vi "Example Threshold - IlluminanceReached Callback.vi"(4 "IlluminanceReached":refnum<user-event>, 5 "Event Data":cluster{"sender":refnum<k24>, "illuminance":i64}, 6 "Control Ref":refnum<k24>, 7 "Event Common Data":T1) -> ()   [LabVIEW 2013]
uses:
  C:/tf/play/labview/Tinkerforge.dll
  Tinkerforge.dll
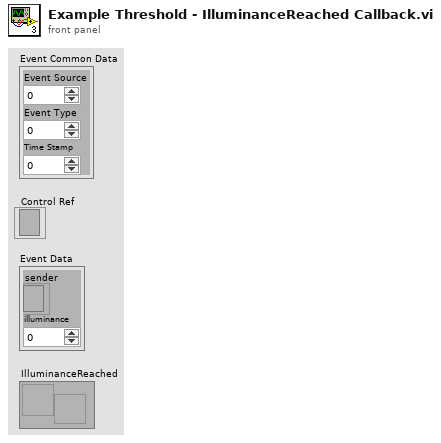
[diagram p1: front panel]
types:
  T1 = cluster{"Event Source":i32, "Event Type":u32, "Time Stamp":u32}
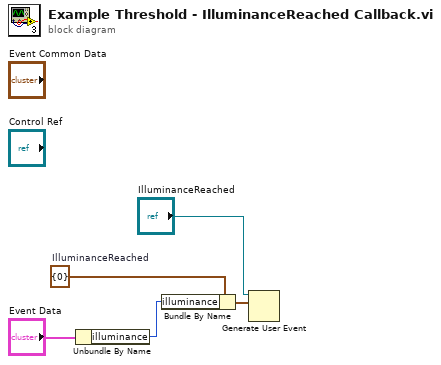
[diagram p0: block diagram]
diagram:
  w4 = cluster{"illuminance":i64} {"illuminance"=0}  # IlluminanceReached
  n1 = Unbundle By Name("Event Data") -> ("illuminance"=w3:i64)
  n2 = Bundle By Name(cluster=w4, "illuminance"=w3) -> (w1:cluster{"illuminance":i64})
  n3 = Generate User Event(user event="IlluminanceReached", event data cluster=w1) -> ()  [unwired: 2 in, 2 out]
